vi "Comm_Write.vi"(8 "error in (no error)":errorcluster, 9 "Text to write":string, 11 "Python":T1) -> (0 "error out":errorcluster)   [LabVIEW 2020]
uses:
  PythonCtrl.ctl
  LabVIEWOpenMV/_subs/Processors.ctl
panel:
  out "result string":string
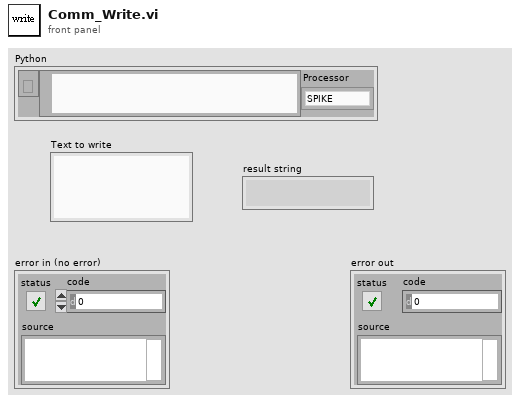
[diagram p1: front panel]
types:
  T1 = typedef "PythonCtrl.ctl" = cluster{"session":refnum<k35>, "PyPath":path, "Processor":T2}
  T2 = typedef "Processors.ctl" = enum16{"SPIKE", "Pi", "Pi_ssh", "OpenMV"}
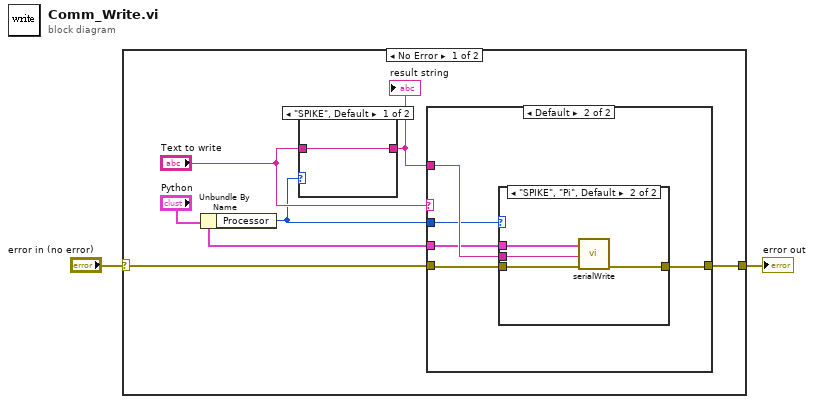
[diagram p0: block diagram]
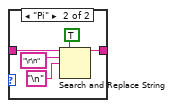
[diagram p2: hidden frame]
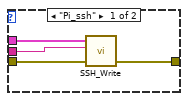
[diagram p4: hidden frame]
diagram:
  n1 = case shown="No Error" "error in (no error)" {
    selector: "error in (no error)" -> [w3 w29]
    tunnel: [w8 w29] -> w2
    frame No Error {
      n2 = Unbundle By Name("Python") -> ("Processor"=w4:T2)
      n3 = case shown="\"SPIKE\", Default" w4 {
        tunnel: "Text to write" -> [w9 w14]
        tunnel: [w9 w13] -> w6
        frame "SPIKE", Default {
        }
        frame "Pi" {
          n4 = Search and Replace String(replace all?=TRUE ("replace all? (F)"), input string=w14, search string="\r\n" ("regular expression"), replace string="\n" ("regular expression")) -> (result string=w13:string)  [unwired: 4 in, 3 out]
        }
      }
      "result string" <- w6
      n5 = case shown="Default" "Text to write" {
        tunnel: w6 -> [_ w20]
        tunnel: w3 -> [w15 w19]
        tunnel: [w15 w18] -> w8
        tunnel: "Python" -> [_ w17]
        tunnel: w4 -> [_ w16]
        frame "" {
        }
        frame Default {
          n6 = case shown="\"SPIKE\", \"Pi\", Default" w16 {
            tunnel: w20 -> [w21 w25]
            tunnel: w19 -> [w24 w28]
            tunnel: [w23 w27] -> w18
            tunnel: w17 -> [w22 w26]
            frame "Pi_ssh" {
              n7 = call "SSH_Write.vi"("error in (no error)"=w24, "Text to write"=w21, "Python"=w22) -> ("error out"=w23:errorcluster)  [unwired: 7 in, 1 out]
            }
            frame "SPIKE", "Pi", Default {
              n8 = call "serialWrite.vi"("error in (no error)"=w28, "text"=w25, "Python"=w26) -> ("error out"=w27:errorcluster)  [unwired: 7 in, 1 out]
            }
          }
        }
      }
    }
    frame Error {
    }
  }
  "error out" <- w2
